vi "Experiment_Write_XML.vi"() -> ()   [LabVIEW 2023]
uses:
  TypeDef/Type_Fit.ctl
  TypeDef/Method_Info.ctl
panel:
  out "Type_Fits":T1[](array[typedef])
  in  "Method_Fit":T2
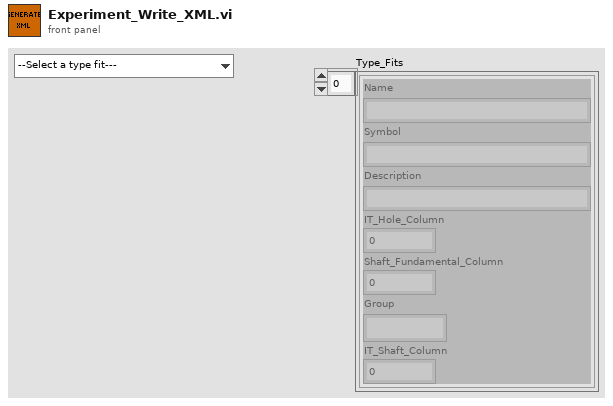
[diagram p1: front panel]
types:
  T1 = typedef "Method_Info.ctl" = cluster{"Name":string, "Symbol":string, "Description":string, "IT_Hole_Column":i32, "Shaft_Fundamental_Column":i32, "Group":string, "IT_Shaft_Column":i32}
  T2 = typedef "Type_Fit.ctl" = enum16{"--Select a type fit---", "Clearance (Loose Running Fit)", "Clearance (Free Running Fit)", "Clearance (Close Running Fit)", "Clearance (Sliding Fit)", "Clearance (Locational Fit)", "Transition (Locational A)", "Transition (Locational B)", "Interference (Locational Fit)", "Interference (Force Fit)", "Interference (Medium Drive Fit)"}
  T3 = enum16{"open", "replace", "create", "open or create", "replace or create", "replace or create with confirmation"}
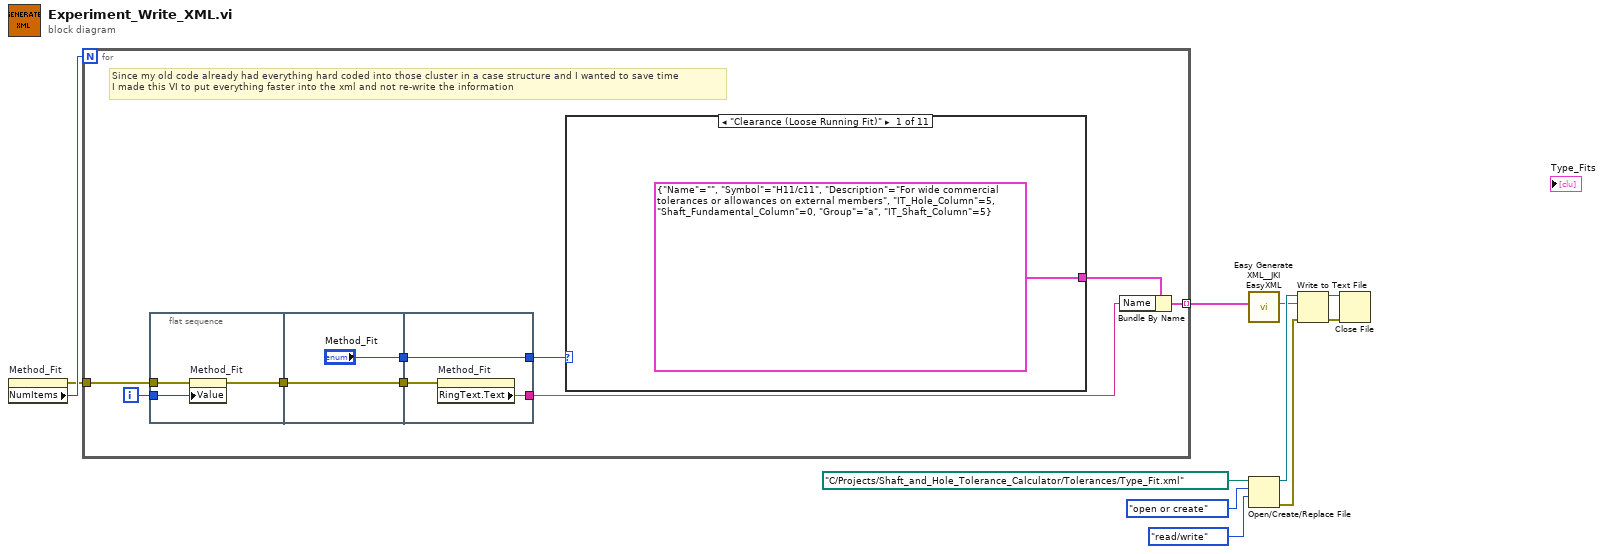
[diagram p0: block diagram]
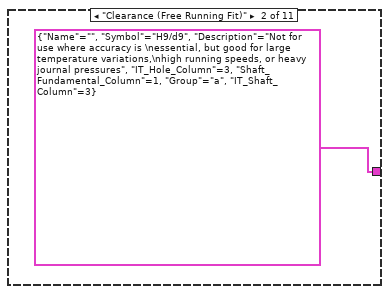
[diagram p2: hidden frame]
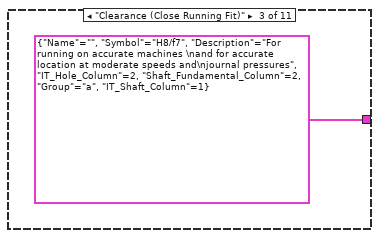
[diagram p3: hidden frame]
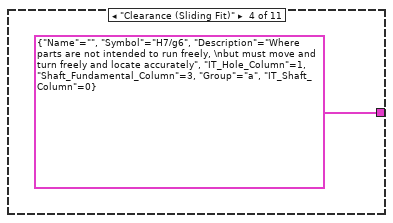
[diagram p4: hidden frame]
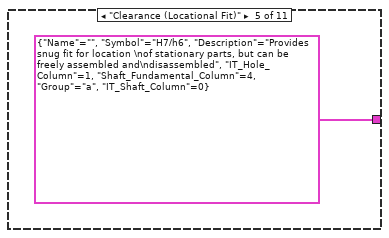
[diagram p5: hidden frame]
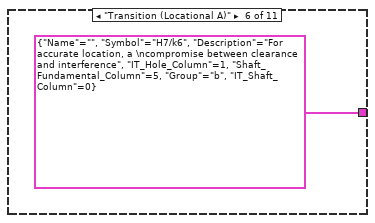
[diagram p6: hidden frame]
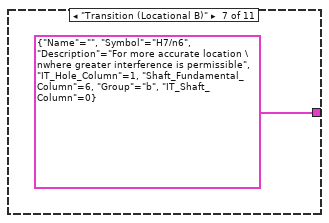
[diagram p7: hidden frame]
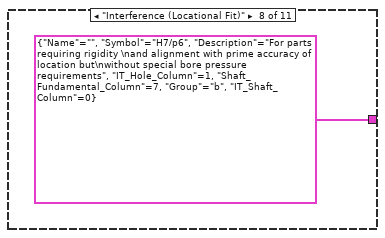
[diagram p8: hidden frame]
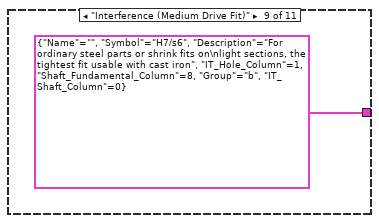
[diagram p9: hidden frame]
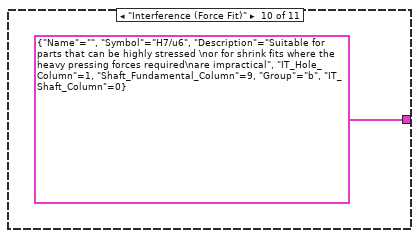
[diagram p10: hidden frame]
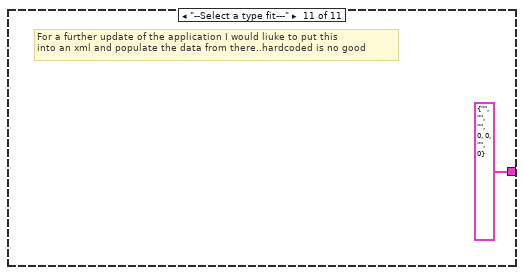
[diagram p11: hidden frame]
diagram:
  n1 = property on="Method_Fit" class="Enum (strict)"() -> (error out=w9:errorcluster, "NumItems"=w11:u32)  [unwired: 2 in, 1 out]
  n2 = for {
    N: w11 -> [_]
    tunnel: [w17] -> w10 mode=indexing
    tunnel: w9 -> [w12]
    i -> [w19]
    # "Since my old code already had everything hard coded into those cluster in a case structure and I wanted to save time\nI made this VI to put everything faster into the xml and not re-write the information"
    n3 = flat-sequence {
      tunnel: w19 -> [w23]
      tunnel: [w22] -> w13
      tunnel: w12 -> [w21]
      tunnel: ["Method_Fit"] -> w16
      tunnel: [w24] -> w14
      tunnel: w13 -> [w24]
      tunnel: [w28] -> w18
      tunnel: w16 -> [w28]
      tunnel: [w27] -> w15
      tunnel: w14 -> [w26]
      frame #0 {
        n4 = property on="Method_Fit" class="Enum (strict)"(error in=w21, "Value"=w23) -> (error out=w22:errorcluster)  [unwired: 1 in, 1 out]
      }
      frame #1 {
      }
      frame #2 {
        n5 = property on="Method_Fit" class="Enum (strict)"(error in=w26) -> ("RingText.Text"=w27:string)  [unwired: 1 in, 2 out]
      }
    }
    n6 = case shown="\"Clearance (Loose Running Fit)\"" w18 {
      tunnel: [T1 {"Name"="", "Symbol"="H11/c11", "Description"="For wide commercial tolerances or allowances on external members", "IT_Hole_Column"=5, "Shaft_Fundamental_Column"=0, "Group"="a", "IT_Shaft_Column"=5} T1 {"Name"="", "Symbol"="H9/d9", "Description"="Not for use where accuracy is \nessential, but good for large temperature variations,\nhigh running speeds, or heavy journal pressures", "IT_Hole_Column"=3, "Shaft_Fundamental_Column"=1, "Group"="a", "IT_Shaft_Column"=3} T1 {"Name"="", "Symbol"="H8/f7", "Description"="For running on accurate machines \nand for accurate location at moderate speeds and\njournal pressures", "IT_Hole_Column"=2, "Shaft_Fundamental_Column"=2, "Group"="a", "IT_Shaft_Column"=1} T1 {"Name"="", "Symbol"="H7/g6", "Description"="Where parts are not intended to run freely, \nbut must move and turn freely and locate accurately", "IT_Hole_Column"=1, "Shaft_Fundamental_Column"=3, "Group"="a", "IT_Shaft_Column"=0} T1 {"Name"="", "Symbol"="H7/h6", "Description"="Provides snug fit for location \nof stationary parts, but can be freely assembled and\ndisassembled", "IT_Hole_Column"=1, "Shaft_Fundamental_Column"=4, "Group"="a", "IT_Shaft_Column"=0} T1 {"Name"="", "Symbol"="H7/k6", "Description"="For accurate location, a \ncompromise between clearance and interference", "IT_Hole_Column"=1, "Shaft_Fundamental_Column"=5, "Group"="b", "IT_Shaft_Column"=0} T1 {"Name"="", "Symbol"="H7/n6", "Description"="For more accurate location \nwhere greater interference is permissible", "IT_Hole_Column"=1, "Shaft_Fundamental_Column"=6, "Group"="b", "IT_Shaft_Column"=0} T1 {"Name"="", "Symbol"="H7/p6", "Description"="For parts requiring rigidity \nand alignment with prime accuracy of location but\nwithout special bore pressure requirements", "IT_Hole_Column"=1, "Shaft_Fundamental_Column"=7, "Group"="b", "IT_Shaft_Column"=0} T1 {"Name"="", "Symbol"="H7/s6", "Description"="For ordinary steel parts or shrink fits on\nlight sections, the tightest fit usable with cast iron", "IT_Hole_Column"=1, "Shaft_Fundamental_Column"=8, "Group"="b", "IT_Shaft_Column"=0} T1 {"Name"="", "Symbol"="H7/u6", "Description"="Suitable for parts that can be highly stressed \nor for shrink fits where the heavy pressing forces required\nare impractical", "IT_Hole_Column"=1, "Shaft_Fundamental_Column"=9, "Group"="b", "IT_Shaft_Column"=0} T1 {"Name"="", "Symbol"="", "Description"="", "IT_Hole_Column"=0, "Shaft_Fundamental_Column"=0, "Group"="", "IT_Shaft_Column"=0}] -> w20
      frame "Clearance (Loose Running Fit)" {
      }
      frame "Clearance (Free Running Fit)" {
      }
      frame "Clearance (Close Running Fit)" {
      }
      frame "Clearance (Sliding Fit)" {
      }
      frame "Clearance (Locational Fit)" {
      }
      frame "Transition (Locational A)" {
      }
      frame "Transition (Locational B)" {
      }
      frame "Interference (Locational Fit)" {
      }
      frame "Interference (Medium Drive Fit)" {
      }
      frame "Interference (Force Fit)" {
      }
      frame "--Select a type fit---" {
        # "For a further update of the application I would liuke to put this \ninto an xml and populate the data from there..hardcoded is no good"
      }
    }
    n7 = Bundle By Name(cluster=w20, "Name"=w15) -> (w17:T1)
  }
  n8 = call <vilib>:"Easy Generate XML__JKI EasyXML.vi"("LabVIEW Data"=w10) -> ("XML String"=w4:string)  [unwired: 9 in, 1 out]
  n9 = Open/Create/Replace File(file path (use dialog)=path "C:/Projects/Shaft_and_Hole_Tolerance_Calculator/Tolerances/Type_Fit.xml", operation (0:open)=T3."open or create", access (0:read/write)=enum16{"read/write", "read-only", "write-only"}."read/write") -> (refnum out=w6:refnum<file>, error out=w5:errorcluster)  [unwired: 3 in, 1 out]
  n10 = Write to Text File(file (use dialog)=w6, text=w4, error in=w5) -> (refnum out=w7:refnum<file>, error out=w8:errorcluster)  [unwired: 1 in, 1 out]
  n11 = Close File(refnum=w7, error in=w8) -> ()  [unwired: 2 out]
